vi "1-Sine Function.vi"() -> ()   [LabVIEW 2014]
panel:
  out "Theta (rad)":dbl
  out "Sine Theta":dbl format="%#_3g"
  in  "Theta (deg)":dbl
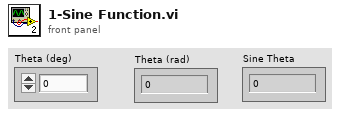
[diagram p1: front panel]
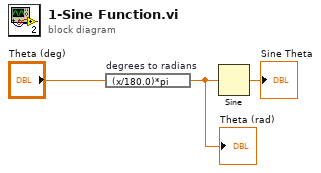
[diagram p0: block diagram]
diagram:
  n1 = expression code="(x/180.0)*pi" "degrees to radians"("Theta (deg)") -> (w1:dbl)
  "Theta (rad)" <- w1
  n2 = Sine(x=w1) -> (sin(x)=→"Sine Theta":dbl)
